vi "write key value.vi"(7 "section":string, 8 "error in (no error)":errorcluster, 9 "value":string, 10 "key":string, 11 "Configuration File in":refnum<class "Configuration File.lvclass">) -> (0 "error out":errorcluster, 3 "Configuration File out":refnum<class "Configuration File.lvclass">)   [LabVIEW 2018, in "Configuration File.lvclass"]
uses:
  Configuration File.lvclass
  Configuration File.lvclass/Configuration File.ctl
  <vilib>/Utility/config.llb/Write Key (String).vi
  <vilib>/Utility/config.llb/NI_LVConfig.lvlib
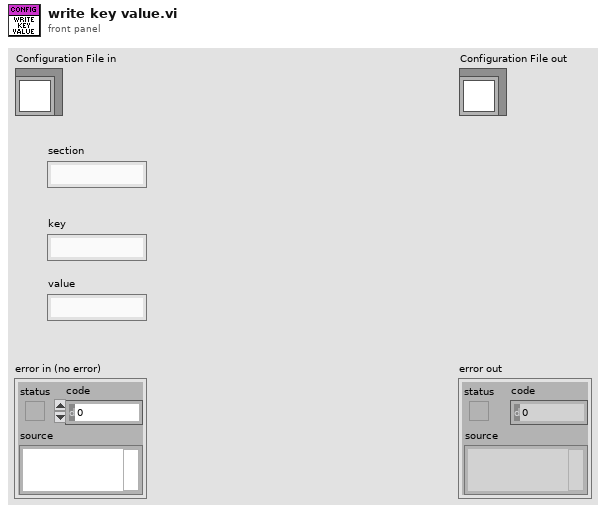
[diagram p1: front panel]
types:
  T1 = typedef "NI_LVConfig.lvlib/Config Data RefNum.ctl" = refnum<k1>
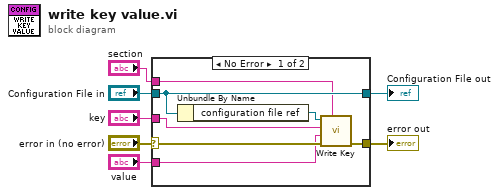
[diagram p0: block diagram]
diagram:
  n1 = case shown="No Error" "error in (no error)" {
    selector: "error in (no error)" -> [w14 w16]
    tunnel: [w13 w16] -> w6
    tunnel: [w12 w15] -> w4
    tunnel: "Configuration File in" -> [w12 w15]
    tunnel: "section" -> [w10 _]
    tunnel: "key" -> [w9 _]
    tunnel: "value" -> [w8 _]
    frame No Error {
      n2 = Unbundle By Name(w12) -> ("configuration file ref"=w11:T1)
      n3 = call-poly <vilib>:"Write Key.vi"("section"=w10, "error in (no error)"=w14, "value"=w8, "key"=w9, "refnum"=w11) -> ("error out"=w13:errorcluster)  [unwired: 4 in, 2 out]
    }
    frame Error {
    }
  }
  "error out" <- w6
  "Configuration File out" <- w4
